vi "Save VI to Previous Version.vi"(9 "版本选择":string(combo), 10 "保存文件的路径":path, 11 "VI路径":path) -> ()   [LabVIEW 2012, in "VIRef.lvlib"]
uses:
  VIRef.lvlib
panel:
  out "错误输出":errorcluster
  in  "错误输入（无错误）":errorcluster
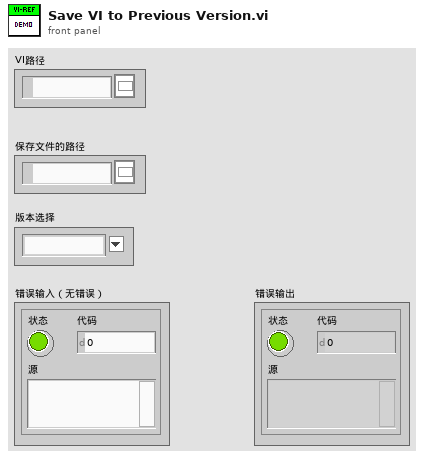
[diagram p1: front panel]
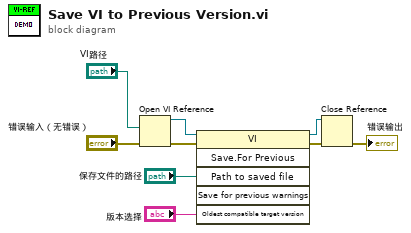
[diagram p0: block diagram]
diagram:
  n1 = Open VI Reference(vi path="VI路径", error in (no error)="错误输入（无错误）") -> (vi reference=w9:refnum<vi>, error out=w7:errorcluster)  [unwired: 4 in]
  n2 = invoke class="VI" method="Save.For Previous"(reference=w9, error in=w7, "Path to saved file"="保存文件的路径", "Oldest compatible target version"="版本选择") -> (reference out=w8:refnum<vi>, error out=w6:errorcluster)  [unwired: 2 in, 4 out]
  n3 = Close Reference(reference=w8, error in (no error)=w6) -> (error out=→"错误输出":errorcluster)
